vi "Serialize.vi"(8 "error in (no error)":errorcluster, 11 "GameRecorder in":refnum<class "GameRecorder.lvclass">) -> (0 "error out":errorcluster, 2 "String":string, 3 "GameRecorder out":refnum<class "GameRecorder.lvclass">)   [LabVIEW 2015, in "TronviewGame.lvlib" / "GameRecorder.lvclass"]
uses:
  GameRecorder.lvclass
  GameRecorder.lvclass/GameRecorder.ctl
  Board/Board.lvclass
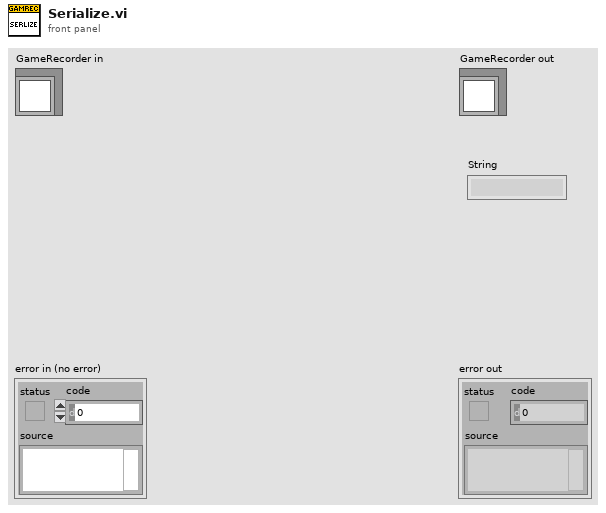
[diagram p1: front panel]
types:
  T1 = typedef "TronVIEWBotAPI.lvlib/MovementDirection.ctl" = enum16{"N", "S", "W", "E"}
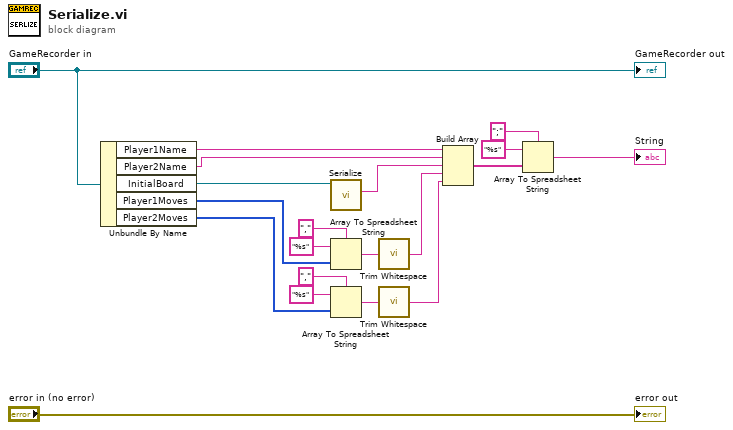
[diagram p0: block diagram]
diagram:
  n1 = Unbundle By Name("GameRecorder in") -> ("Player1Name"=w18:string, "Player2Name"=w17:string, "InitialBoard"=w16:refnum<class "Board.lvclass">, "Player1Moves"=w13:T1[], "Player2Moves"=w8:T1[])
  n2 = call "Serialize.vi"("Board in"=w16) -> ("SerializedBoard"=w15:string)  [unwired: 8 in, 2 out]
  n3 = Array To Spreadsheet String(delimiter (Tab)=",", array=w13, 3:"%s" ("format string")) -> (spreadsheet string=w11:string)
  n4 = Array To Spreadsheet String(delimiter (Tab)=",", array=w8, 3:"%s" ("format string")) -> (spreadsheet string=w7:string)
  n5 = call <vilib>:"Trim Whitespace.vi"("string"=w11) -> ("trimmed string"=w2:string)  [unwired: 1 in]
  n6 = call <vilib>:"Trim Whitespace.vi"("string"=w7) -> ("trimmed string"=w1:string)  [unwired: 1 in]
  n7 = Build Array(w18, w17, w15, w2, w1) -> (w4:string[])
  n8 = Array To Spreadsheet String(delimiter (Tab)=";", array=w4, 3:"%s" ("format string")) -> (spreadsheet string=→"String":string)
  "error out" <- "error in (no error)"
  "GameRecorder out" <- "GameRecorder in"
